vi "Add Item.vi"(4 "Pattern":string, 5 "Path":path, 7 "error in":errorcluster, 8 "Path to start the search":path, 9 "Parent Tag":string, 10 "Tree In":refnum<vi>) -> (0 "error out":errorcluster, 1 "Files Found":path[](array[path]), 2 "Folders Found":path[](array[path]), 3 "Tree Out":refnum<vi>)   [LabVIEW 2011]
doc: "This VI populates the tree control with the folders and their respective subfolders and files. \nIf Pattern to search control has a valid file type extension, only those files will be displayed."
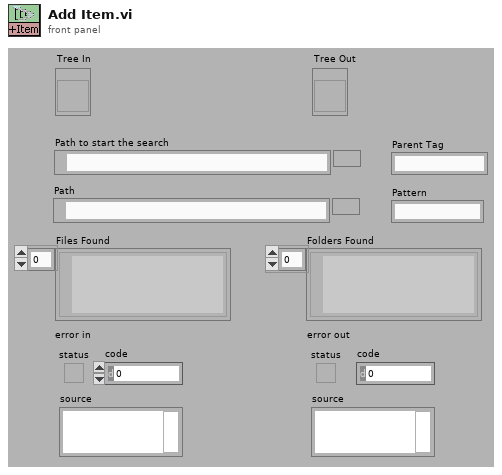
[diagram p1: front panel]
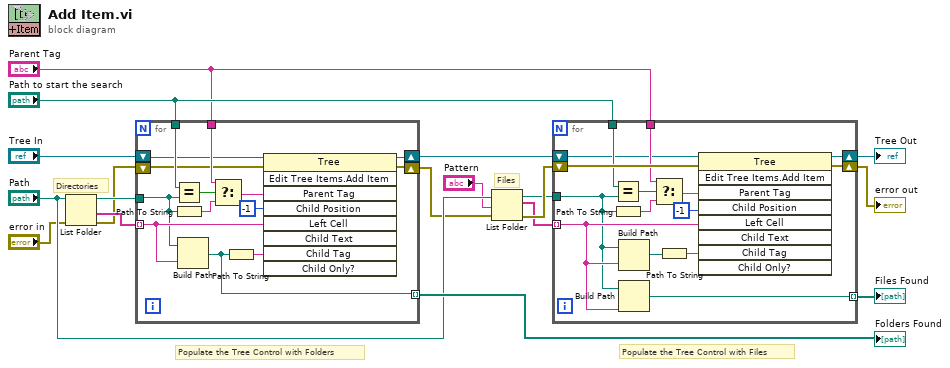
[diagram p0: block diagram]
diagram:
  # "Populate the Tree Control with Files"
  # "Populate the Tree Control with Folders"
  # "Files"
  # "Directories"
  n1 = List Folder(path="Path", error in="error in") -> (path out=w17:path, folder names=w13:string[], error out=w5:errorcluster)  [unwired: 2 in, 1 out]
  n2 = for {
    tunnel: w17 -> [w24]
    tunnel: [w30] -> w16 mode=indexing
    tunnel: w13 -> [w31] mode=indexing
    tunnel: "Parent Tag" -> [w26]
    tunnel: "Path to start the search" -> [w23]
    shift-right: [w21] -> w6
    shift-left: w5 -> [w20]
    shift-right: [w19] -> w2
    shift-left: "Tree In" -> [w22]
    n3 = Equal?(x=w23, y=w24) -> (x = y?=w28:bool)
    n4 = Path To String(path=w24) -> (string=w27:string)
    n5 = Build Path(base path=w24, name or relative path=w31) -> (appended path=w30:path)
    n6 = Select(t=w26, s=w28, f=w27) -> (s? t:f=w25:string)
    n7 = Path To String(path=w30) -> (string=w29:string)
    n8 = invoke on="Invoke Node" class="Tree" method="Edit Tree Items.Add Item"(reference=w22, error in=w20, "Parent Tag"=w25, "Child Position"=-1 ("Child Posn"), "Left Cell"=w31, "Child Tag"=w29) -> (reference out=w19:refnum<vi>, error out=w21:errorcluster)  [unwired: 3 in, 7 out]
  }
  "Folders Found" <- w16
  n9 = List Folder(path="Path", pattern="Pattern", error in=w6) -> (path out=w8:path, filenames=w7:string[], error out=w9:errorcluster)  [unwired: 1 in, 1 out]
  n10 = for {
    tunnel: [w47] -> w4 mode=indexing
    tunnel: w7 -> [w41] mode=indexing
    tunnel: "Parent Tag" -> [w38]
    tunnel: w8 -> [w35]
    tunnel: "Path to start the search" -> [w39]
    shift-right: [w45] -> w11
    shift-left: w9 -> [w46]
    shift-right: [w33] -> w1
    shift-left: w2 -> [w34]
    n11 = Equal?(x=w39, y=w35) -> (x = y?=w40:bool)
    n12 = Path To String(path=w35) -> (string=w37:string)
    n13 = Build Path(base path=w35, name or relative path=w41) -> (appended path=w43:path)
    n14 = Build Path(base path=w35, name or relative path=w41) -> (appended path=w47:path)
    n15 = Select(t=w38, s=w40, f=w37) -> (s? t:f=w36:string)
    n16 = Path To String(path=w43) -> (string=w42:string)
    n17 = invoke on="Invoke Node" class="Tree" method="Edit Tree Items.Add Item"(reference=w34, error in=w46, "Parent Tag"=w36, "Child Position"=-1 ("Child Posn"), "Left Cell"=w41, "Child Tag"=w42) -> (reference out=w33:refnum<vi>, error out=w45:errorcluster)  [unwired: 3 in, 7 out]
  }
  "Files Found" <- w4
  "error out" <- w11
  "Tree Out" <- w1
